vi "模拟输入_有限.vi"() -> ()   [LabVIEW 2013]
doc: "This example demonstrates how to acquire a finite amount of data."
uses:
  <userlib>/ArtDAQ/_SubVI/ArtDAQ_CreateAIVoltageChan.vi
  <userlib>/ArtDAQ/_SubVI/ArtDAQ_CfgSampClkTiming.vi
  <userlib>/ArtDAQ/_SubVI/ArtDAQ_Read Analog DBL NChan NSamp.vi
  <userlib>/ArtDAQ/_SubVI/ArtDAQ_CfgDigEdgeStartTrig.vi
  <userlib>/ArtDAQ/_SubVI/ArtDAQ_CfgAnlgEdgeStartTrig.vi
panel:
  in  "触发模式":enum32{"无触发", "数字边沿", "模拟边沿"}(tab)
  in  "触发源":string="/Dev1/PFI1"
  in  "触发边沿":i32(ring)=10280 items=["上升"=10280, "下降"=10171]
  in  "触发电平(V)":dbl
  in  "触发源":string(combo)="Dev1/ai0"
  in  "斜率":i32(ring)=10280 items=["上升"=10280, "下降"=10171]
  out "波形图":dbl[][](graph)
  in  "采样速率":dbl=10000.0 format="%#_13g"
  in  "每通道采样点数":i32=1000
  in  "接线端配置":i32(ring)=-1 items=["默认"=-1, "单端"=10083, "非参考单端"=10078, "差分"=10106, "伪差分"=12529]
  in  "最小值(V)":dbl=-10.0 format="%#_13g"
  in  "最大值(V)":dbl=10.0 format="%#_13g"
  in  "物理通道":string(combo)="Dev1/ai0"
  out "错误":errorcluster
  # "通道属性"
  # "定时"
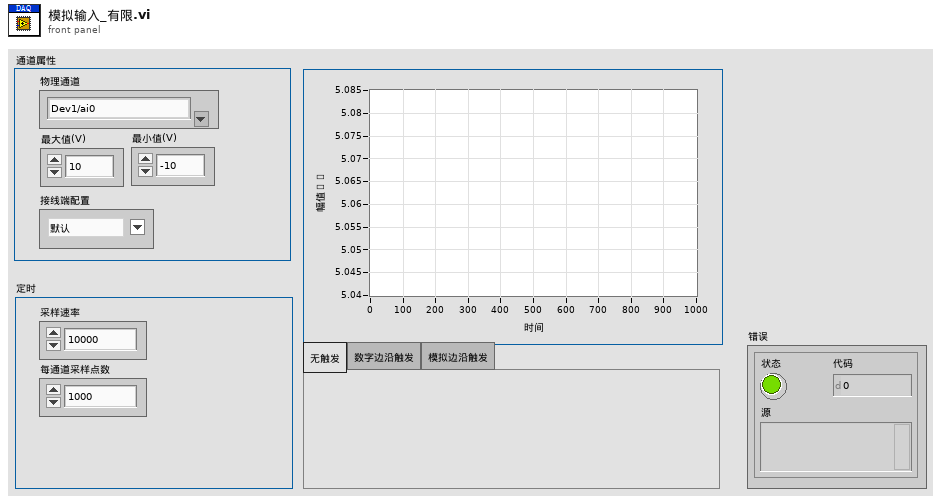
[diagram p1: front panel]
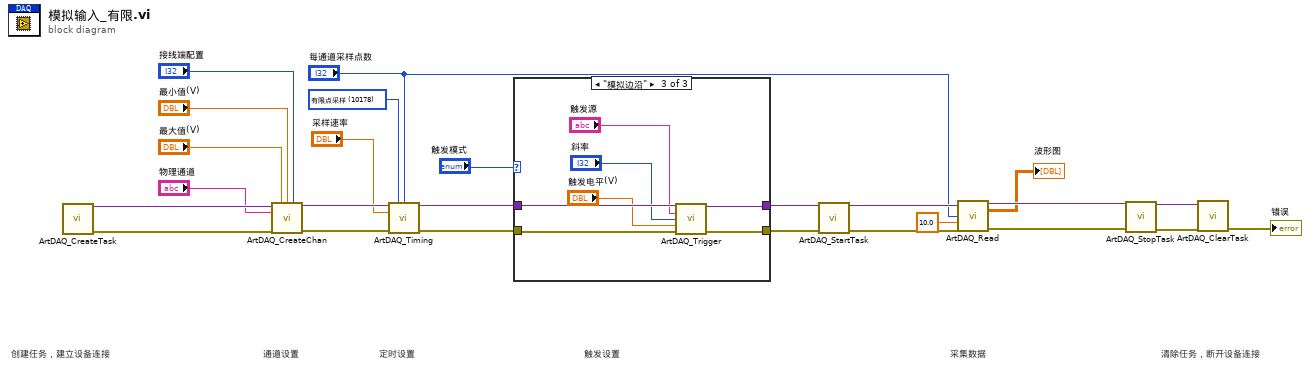
[diagram p0: block diagram]
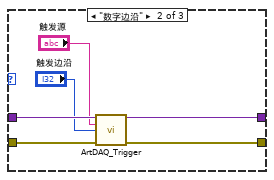
[diagram p3: hidden frame]
diagram:
  w19 = 10178 items=["有限点采样"=10178, "连续采样"=10123] ("SampleMode")
  # "清除任务，断开设备连接"
  # "采集数据"
  # "触发设置"
  # "定时设置"
  # "通道设置"
  # "创建任务，建立设备连接"
  n1 = call <userlib>:"ArtDAQ_CreateTask.vi"() -> ("任务句柄"=w13:variant, "错误输出"=w25:errorcluster)  [unwired: 14 in]
  n2 = call-poly <userlib>:"ArtDAQ_CreateChan.vi"("任务句柄"=w13, "最大值"="最大值(V)", "最小值"="最小值(V)", "接线端配置"="接线端配置", "物理通道"="物理通道", "错误输入"=w25) -> ("任务句柄"=w21:variant, "错误输出"=w20:errorcluster)  [unwired: 8 in]
  n3 = call-poly <userlib>:"ArtDAQ_Timing.vi"("任务句柄"=w21, "采样模式"=w19, "每通道采样数"="每通道采样点数", "采样率"="采样速率", "错误输入"=w20) -> ("任务句柄"=w8:variant, "错误输出"=w6:errorcluster)  [unwired: 9 in]
  n4 = case shown="\"模拟边沿\"" "触发模式" {
    tunnel: w8 -> [w27 w33 w40]
    tunnel: [w27 w32 w39] -> w7
    tunnel: w6 -> [w26 w30 w37]
    tunnel: [w26 w31 w38] -> w5
    frame "无触发", Default {
    }
    frame "数字边沿" {
      n5 = call-poly <userlib>:"ArtDAQ_Trigger.vi"("任务句柄"=w33, "触发源"="触发源", "边沿"="触发边沿", "错误输入"=w30) -> ("任务句柄"=w32:variant, "错误输出"=w31:errorcluster)  [unwired: 10 in]
    }
    frame "模拟边沿" {
      n6 = call-poly <userlib>:"ArtDAQ_Trigger.vi"("任务句柄"=w40, "触发源"="触发源", "斜率"="斜率", "触发电平"="触发电平(V)", "错误输入"=w37) -> ("任务句柄"=w39:variant, "错误输出"=w38:errorcluster)  [unwired: 9 in]
    }
  }
  n7 = call <userlib>:"ArtDAQ_StartTask.vi"("任务句柄"=w7, "错误输入"=w5) -> ("任务句柄"=w16:variant, "错误输出"=w15:errorcluster)  [unwired: 12 in]
  n8 = call-poly <userlib>:"ArtDAQ_Read.vi"("任务句柄"=w16, "每通道采样数"="每通道采样点数", "超时s"=10.0 ("Timeout"), "错误输入"=w15) -> ("任务句柄"=w12:variant, "数据"=→"波形图":dbl[][], "错误输出"=w11:errorcluster)  [unwired: 8 in, 1 out]
  n9 = call <userlib>:"ArtDAQ_StopTask.vi"("任务句柄"=w12, "错误输入"=w11) -> ("任务句柄"=w10:variant, "错误输出"=w9:errorcluster)  [unwired: 12 in]
  n10 = call <userlib>:"ArtDAQ_ClearTask.vi"("任务句柄"=w10, "错误输入"=w9) -> ("错误输出"=→"错误":errorcluster)  [unwired: 13 in]
